vi "FPGA - Current Mode.vi"() -> ()   [LabVIEW 2018]
uses:
  <vilib>/rvi/Analysis/control/PID/Typedef/niFpgaPID_PIGains.ctl
  <vilib>/rvi/Analysis/control/PID/Typedef/niFpgaPID_OutputRange.ctl
  <vilib>/rvi/Emulation/niFpgaGetClockAttributes.vi
  <vilib>/rvi/Emulation/niFpgaSctlEmulationGetInTimedLoop.vi
  <vilib>/rvi/Emulation/niFpgaEmulationReportErrorSimple.vi
  <vilib>/rvi/eio/common/nirviEmuTemplateMethod_errors.vi
  <vilib>/rvi/Analysis/control/PID/SubVIs/niFpgaPID_PIWrapper.vi
  <vilib>/rvi/Emulation/niFpgaCriticalErrorInLSC.vi
  <vilib>/rvi/interface/RandomDataEmulation/niFpgaRandomDataHandleErrors.vi
  <vilib>/eio/EIONode/EIONode.xnode
  <vilib>/rvi/DataTransferAndStorage/Container/XNode/niFpgaContainer.xnode
  <vilib>/rvi/interface/RandomDataEmulation/nirviRandomDataFpgaReadWriteTemplate.vi
panel:
  in  "Numeric Control":u16
  in  "PID":bool
  in  "Slow\nLoop \nRate \n(us)":u32 caption="PID Loop Rate (us)"
  out "Sense resistor voltage":i16
  in  "Measure":bool
  in  "Sense\nLoop \nRate \n(us)":u32 caption="Sense Loop Rate (us)"
  in  "Amplifier\nOn/Off":bool
  out "PID Error (V)":sgl
  out "PID Output (V)":u16
  in  "output range":T1={"output high (Inf)"=inf, "output low (-Inf)"=-inf}
  in  "gains":T2 {"proportional gain" step=0.125}
  out "Capacitance\nProbe (V)":sgl
  out "Capacitance\nProbe (um)":sgl
  in  "PID\nLoop \nRate \n(us)":u32 caption="PID Loop Rate (us)"
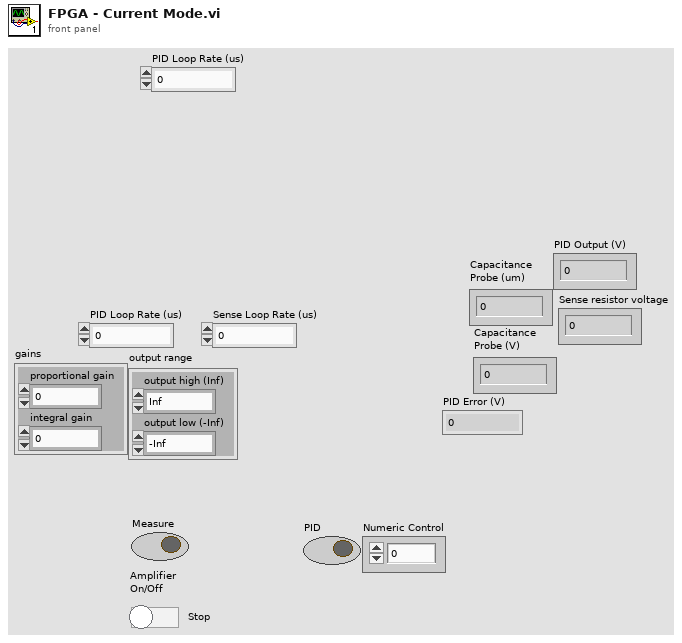
[diagram p1: front panel]
types:
  T1 = typedef "niFpgaPID_OutputRange.ctl" = cluster{"output high (Inf)":sgl, "output low (-Inf)":sgl}
  T2 = typedef "niFpgaPID_PIGains.ctl" = cluster{"proportional gain":sgl, "integral gain":sgl}
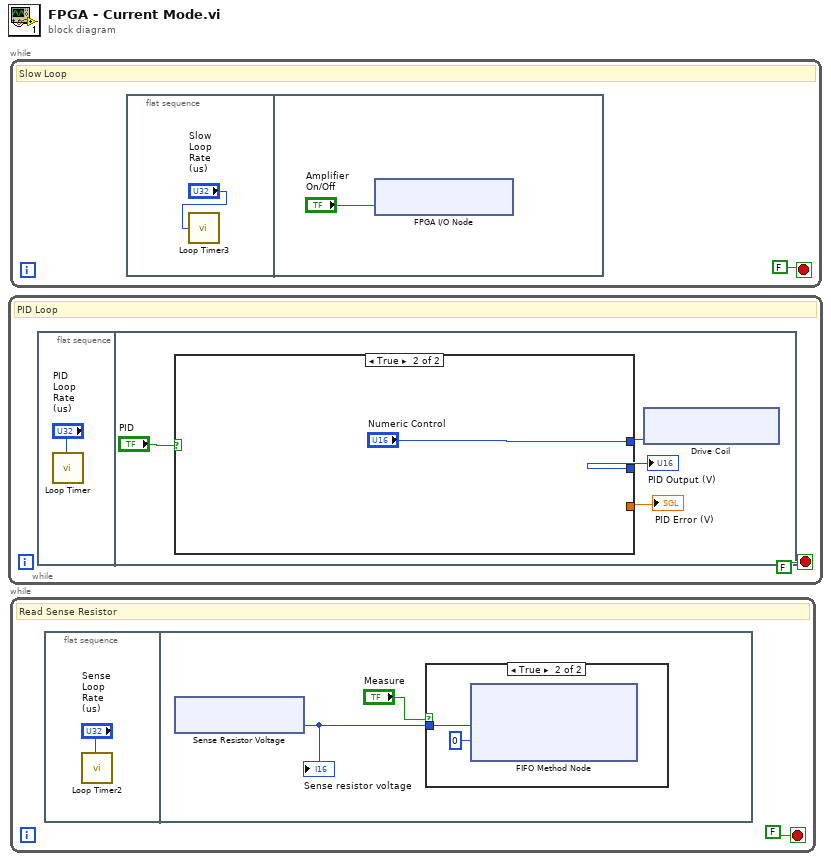
[diagram p0: block diagram]
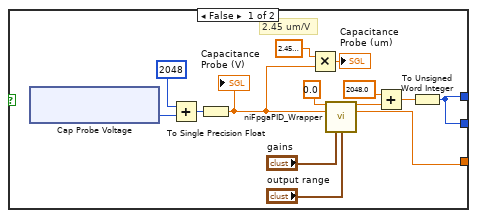
[diagram p3: hidden frame]
diagram:
  n1 = while {
    stop <- FALSE stop-if-true
    # "PID Loop"
    n2 = flat-sequence {
      frame #0 {
        n3 = call "Loop Timer"("Count(uSec)"="PID\nLoop \nRate \n(us)") -> ()  [unwired: 1 out]
      }
      frame #1 {
        n4 = case shown="True" "PID" {
          tunnel: [w7 "Numeric Control"] -> w6
          tunnel: [w8 _] -> w5
          tunnel: [w7 _] -> w4
          frame False {
            # "2.45 um/V"
            n5 = xnode "Cap Probe Voltage"() -> ("ConnectorC/AI0"=w20:i16)  [unwired: 1 in, 1 out]
            n6 = Add(x=i16 2048, y=w20) -> (x+y=w17:i16)
            n7 = To Single Precision Float(number=w17) -> (single precision float=w12:sgl)
            "Capacitance\nProbe (V)" <- w12
            n8 = Multiply(x=sgl 2.45 ("y"), y=w12) -> (x*y=→"Capacitance\nProbe (um)":sgl)
            n9 = call-poly <vilib>:"niFpgaPID_Wrapper.vi"("setpoint"=sgl 0.0, "process variable"=w12, "gains"="gains", "output range"="output range") -> ("output"=w11:sgl, "error"=w8:sgl)  [unwired: 9 in, 1 out]
            n10 = Add(x=sgl 2048.0, y=w11) -> (x+y=w9:sgl)
            n11 = To Unsigned Word Integer(number=w9) -> (unsigned 16bit integer=w7:u16)
          }
          frame True {
          }
        }
        "PID Output (V)" <- w4
        "PID Error (V)" <- w5
        n12 = xnode "Drive Coil"("ConnectorA/AO1"=w6) -> ()  [unwired: 1 in, 1 out]
      }
    }
  }
  n13 = while {
    stop <- FALSE stop-if-true
    # "Slow Loop"
    n14 = flat-sequence {
      frame #0 {
        n15 = call "Loop Timer3"("Count(uSec)"="Slow\nLoop \nRate \n(us)") -> ()  [unwired: 1 out]
      }
      frame #1 {
        n16 = xnode "FPGA I/O Node"("ConnectorA/DIO9"="Amplifier\nOn/Off") -> ()  [unwired: 1 in, 1 out]
      }
    }
  }
  n17 = while {
    stop <- FALSE stop-if-true
    # "Read Sense Resistor"
    n18 = flat-sequence {
      frame #0 {
        n19 = call "Loop Timer2"("Count(uSec)"="Sense\nLoop \nRate \n(us)") -> ()  [unwired: 1 out]
      }
      frame #1 {
        n20 = xnode "Sense Resistor Voltage"() -> ("ConnectorC/AI1"=w28:i16)  [unwired: 1 in, 1 out]
        "Sense resistor voltage" <- w28
        n21 = case shown="True" "Measure" {
          tunnel: w28 -> [_ w30]
          frame False {
          }
          frame True {
            n22 = xnode ("FIFO Method Node")("Element"=w30, "Timeout"=0) -> ()  [unwired: 1 in, 2 out]
          }
        }
      }
    }
  }
